vi "test5.vi"() -> ()   [LabVIEW 2020]
uses:
  bee2abb7-c490-4ad6-bfc0-30ed72578e14.vi
panel:
  out "Array":cluster{"x":dbl, "y":dbl}[](array[cluster])
  in  "input variable":dbl=5.5 format="%#_13g"
  out "XY Graph":cluster{dbl[], dbl[]}(graph)
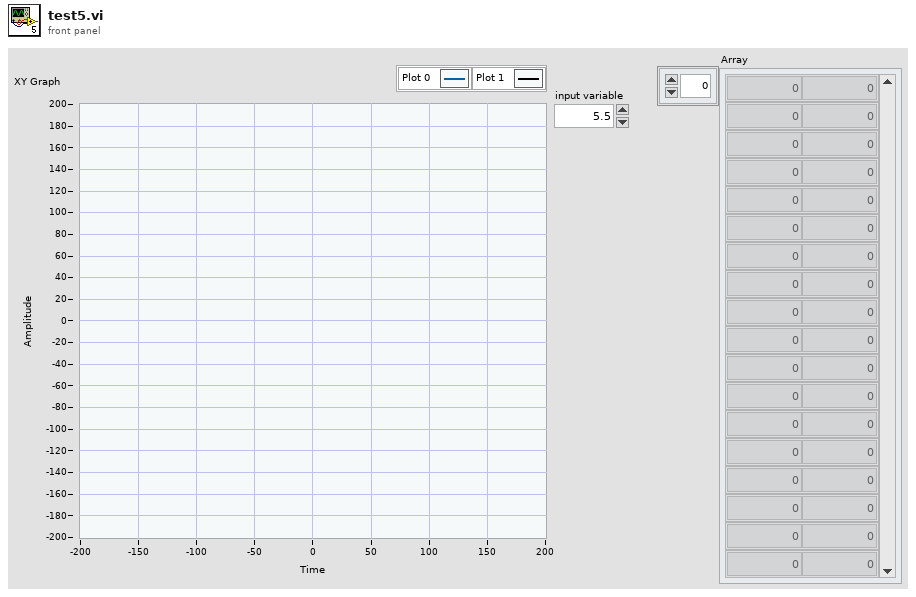
[diagram p1: front panel]
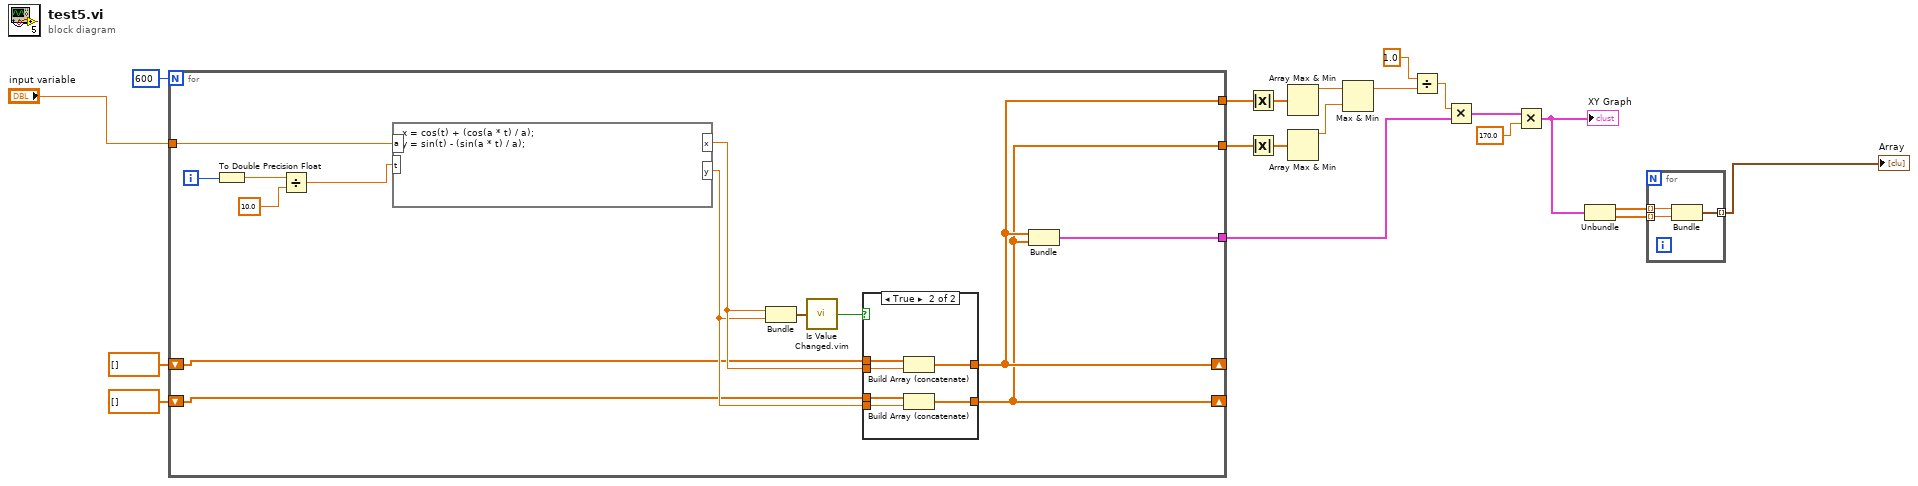
[diagram p0: block diagram]
diagram:
  n1 = for {
    N: 600 -> [_]
    tunnel: "input variable" -> [w34]
    shift-right: [w22] -> _
    shift-left: dbl[] [] -> [w29]
    shift-right: [w21] -> _
    shift-left: dbl[] [] -> [w28]
    tunnel: [w27] -> w7
    tunnel: [w22] -> w16
    tunnel: [w21] -> w15
    i -> [w26]
    n2 = To Double Precision Float(number=w26) -> (double precision float=w25:dbl)
    n3 = Divide(x=w25, y=10.0) -> (x/y=w23:dbl)
    n4 = formula code="x = cos(t) + (cos(a * t) / a);\ny = sin(t) - (sin(a * t) / a);"("a"=w34, "t"=w23) -> ("x"=w31:dbl, "y"=w30:dbl)
    n5 = Bundle("x"=w31, "y"=w30) -> (w33:cluster{"x":dbl, "y":dbl})  [unwired: 1 in]
    n6 = call "Is Value Changed.vim"("value"=w33) -> ("changed or first call?"=w32:bool)
    n7 = case shown="True" w32 {
      tunnel: w31 -> [_ w42]
      tunnel: w30 -> [_ w41]
      tunnel: [w36 w40] -> w22
      tunnel: [w35 w39] -> w21
      tunnel: w29 -> [w36 w38]
      tunnel: w28 -> [w35 w37]
      frame False {
      }
      frame True {
        n8 = Build Array (concatenate)(w38, w42) -> (w40:dbl[])
        n9 = Build Array (concatenate)(w37, w41) -> (w39:dbl[])
      }
    }
    n10 = Bundle(w22, w21) -> (w27:cluster{dbl[], dbl[]})  [unwired: 1 in]
  }
  n11 = Absolute Value(x=w16) -> (abs(x)=w14:dbl[])
  n12 = Absolute Value(x=w15) -> (abs(x)=w13:dbl[])
  n13 = Array Max & Min(array=w14) -> (max value=w12:dbl)  [unwired: 3 out]
  n14 = Array Max & Min(array=w13) -> (max value=w11:dbl)  [unwired: 3 out]
  n15 = Max & Min(x=w12, y=w11) -> (max(x,y)=w10:dbl)  [unwired: 1 out]
  n16 = Divide(x=1.0, y=w10) -> (x/y=w8:dbl)
  n17 = Multiply(x=w8, y=w7) -> (x*y=w6:cluster{dbl[], dbl[]})
  n18 = Multiply(x=w6, y=170.0 ("x")) -> (x*y=w4:cluster{dbl[], dbl[]})
  "XY Graph" <- w4
  n19 = Unbundle(w4) -> (w3:dbl[], w2:dbl[])
  n20 = for {
    tunnel: w3 -> [w45] mode=indexing
    tunnel: w2 -> [w44] mode=indexing
    tunnel: [w43] -> w1 mode=indexing
    n21 = Bundle("x"=w45, "y"=w44) -> (w43:cluster{"x":dbl, "y":dbl})  [unwired: 1 in]
  }
  "Array" <- w1
